vi "ELCN100 Project.vi"() -> ()   [LabVIEW 2021]
uses:
  <vilib>/Analysis/4window.llb/windowTd.ctl
  <vilib>/measure/maspectr.llb/FFT Power Spectrum and PSD for 1 Chan.vi
  <vilib>/measure/NI_MAPro.lvlib
  <vilib>/measure/NI_MABase.lvlib
  <vilib>/Analysis/NI_AALPro.lvlib
panel:
  in  "Noise Amplitude":dbl(knob) scale=0.0..10.0
  in  "Signal type":enum16{"Sine", "Square", "Triangle", "Sawtooth"}(ring)
  out "Time Domain":waveform(dbl)(graph)
  in  "stop":bool
  in  "Frequency":dbl(knob) scale=0.0..500.0 scale format="%^#_3g"
  in  "Averaging parameters":T1={"averaging mode"=enum."No averaging", "weighting mode"=enum."Exponential", "number of averages"=10} {"number of averages" min=1}
  in  "dB On (F)":bool
  in  "window":T2=1 items=["Rectangle"=0, "Hanning"=1, "Hamming"=2, "Blackman-Harris"=3, "Exact Blackman"=4, "Blackman"=5, "Flat Top"=6, "4 Term B-Harris "=7, "7 Term B-Harris"=8, "Low Sidelobe"=9, "Blackman Nuttall"=11, "Triangle"=30, "Bartlett-Hanning"=31, "Bohman"=32, "Parzen"=33, "Welch"=34, "Kaiser"=60, "Dolph-Chebyshev"=61, "Gaussian"=62]
  out "Frequency Domain":cluster{"f0":dbl, "df":dbl, "magnitude":dbl[]}(graph)
  in  "Amplitude":dbl
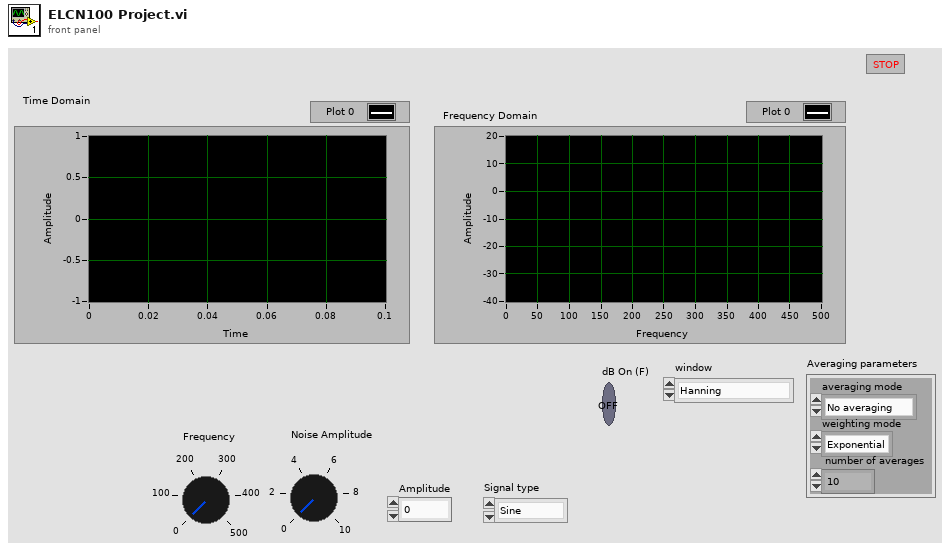
[diagram p1: front panel]
types:
  T1 = cluster{"averaging mode":enum16{"No averaging", "Vector averaging", "RMS averaging", "Peak hold"}, "weighting mode":enum16{"Linear", "Exponential"}, "number of averages":u32}
  T2 = typedef "NI_AALPro.lvlib/windowTd.ctl" = u32
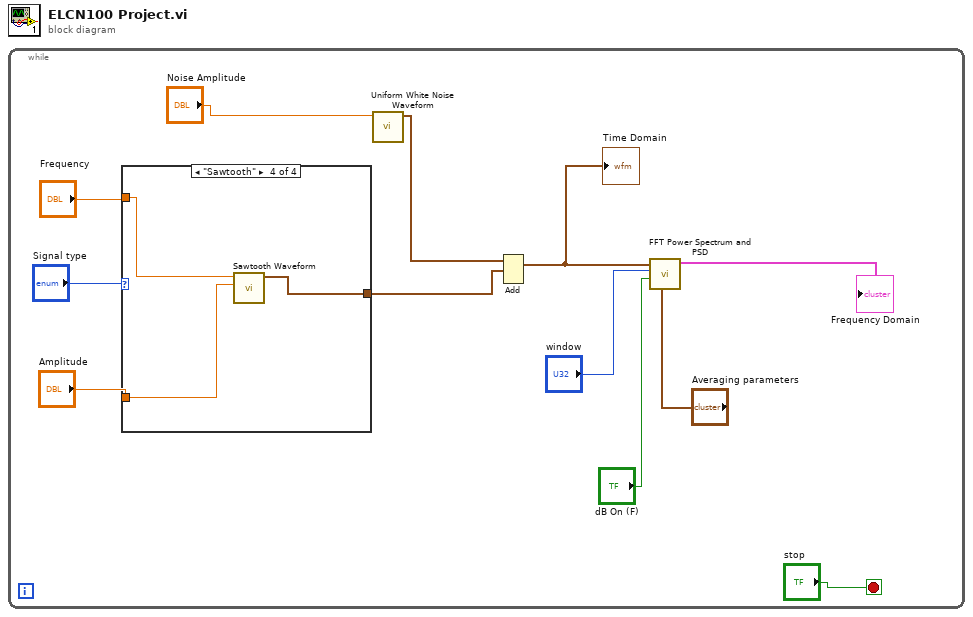
[diagram p0: block diagram]
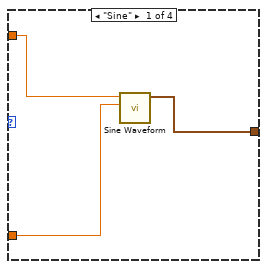
[diagram p2: hidden frame]
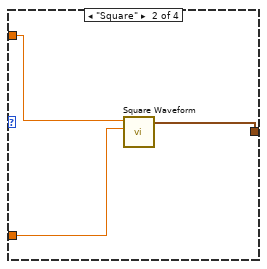
[diagram p3: hidden frame]
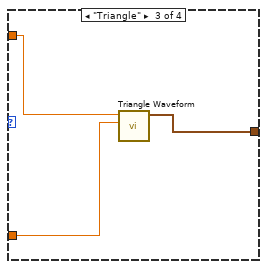
[diagram p4: hidden frame]
diagram:
  n1 = while {
    stop <- "stop" stop-if-true
    n2 = case shown="\"Sawtooth\"" "Signal type" {
      tunnel: "Frequency" -> [w15 w18 w21 w24]
      tunnel: "Amplitude" -> [w14 w17 w20 w23]
      tunnel: [w13 w16 w19 w22] -> w3
      frame "Sine" {
        n3 = call <vilib>:"Sine Waveform.vi"("amplitude"=w14, "frequency"=w15) -> ("signal out"=w13:waveform(dbl))  [unwired: 8 in, 1 out]
      }
      frame "Square" {
        n4 = call <vilib>:"Square Waveform.vi"("amplitude"=w17, "frequency"=w18) -> ("signal out"=w16:waveform(dbl))  [unwired: 8 in, 1 out]
      }
      frame "Triangle" {
        n5 = call <vilib>:"Triangle Waveform.vi"("amplitude"=w20, "frequency"=w21) -> ("signal out"=w19:waveform(dbl))  [unwired: 8 in, 1 out]
      }
      frame "Sawtooth" {
        n6 = call <vilib>:"Sawtooth Waveform.vi"("amplitude"=w23, "frequency"=w24) -> ("signal out"=w22:waveform(dbl))  [unwired: 8 in, 1 out]
      }
    }
    n7 = call <vilib>:"Uniform White Noise Waveform.vi"("amplitude"="Noise Amplitude") -> ("signal out"=w5:waveform(dbl))  [unwired: 9 in, 1 out]
    n8 = Add(1:w3, 2:w5) -> (0:w4:waveform(dbl))  [unwired: 1 in, 1 out]
    "Time Domain" <- w4
    n9 = call-poly <vilib>:"FFT Power Spectrum and PSD.vi"("averaging parameters"="Averaging parameters", "dB On (F)"="dB On (F)", "window"="window", "time signal"=w4) -> ("Power Spectrum / PSD"=→"Frequency Domain":cluster{"f0":dbl, "df":dbl, "magnitude":dbl[]})  [unwired: 4 in, 3 out]
  }
